vi "RT Status.vi"() -> ()   [LabVIEW 2019]
panel:
  out "rt queue":refnum<queue>
  out "status":string
  out "error out":errorcluster
  out "state":enum16{"connect", "run", "close"}(ring)
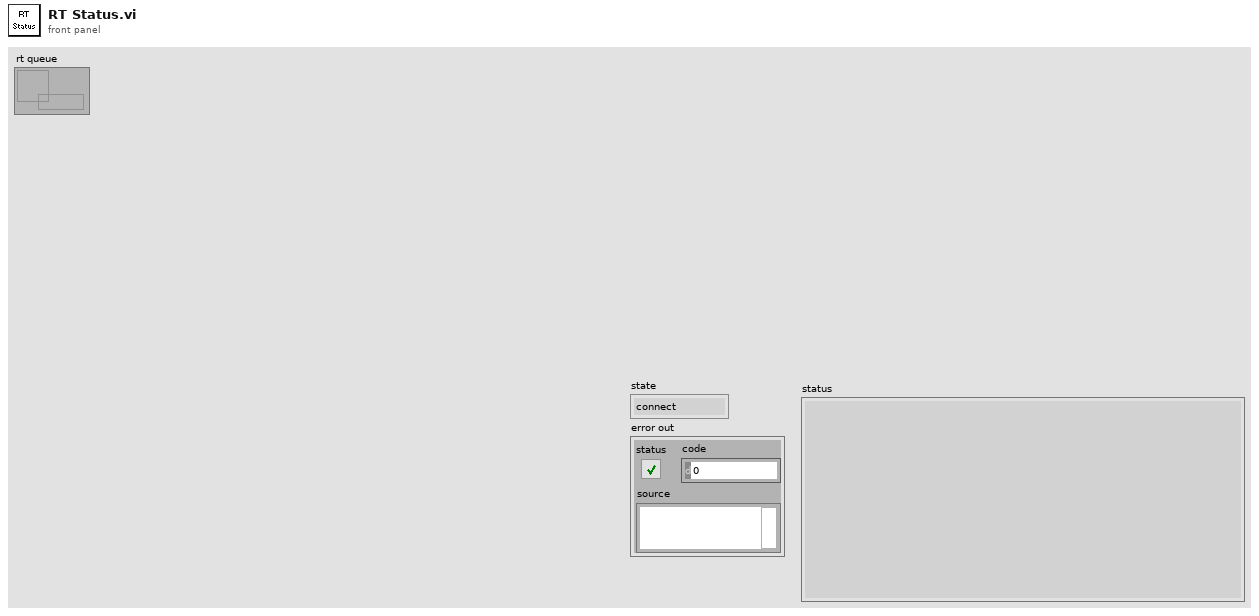
[diagram p1: front panel]
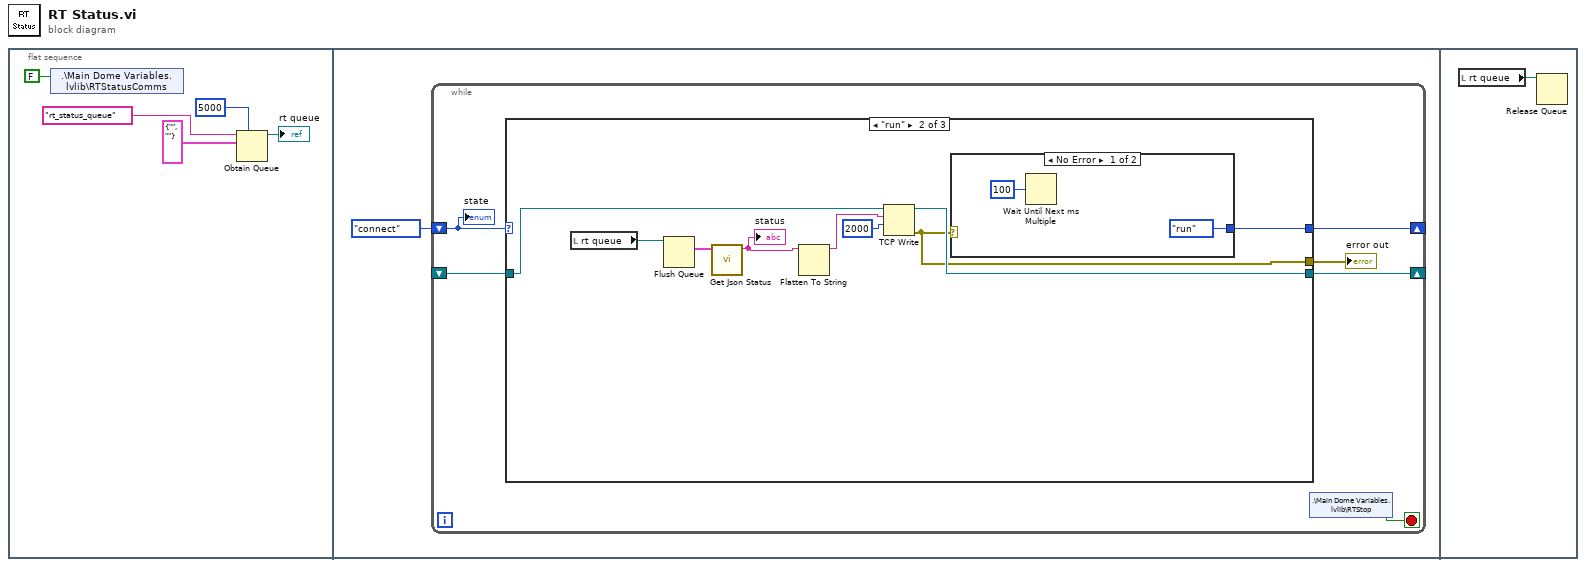
[diagram p0: block diagram]
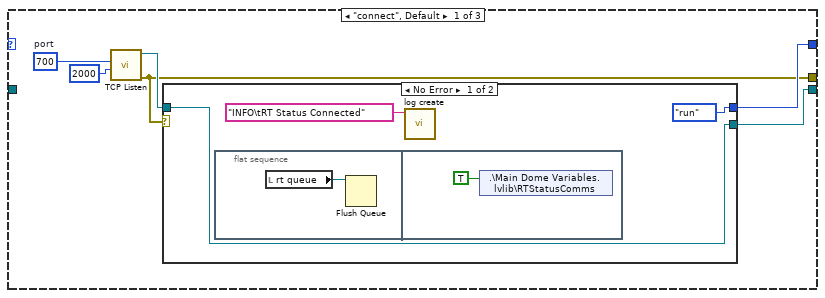
[diagram p2: hidden frame]
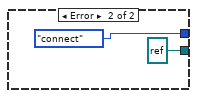
[diagram p3: hidden frame]
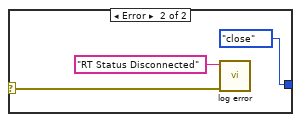
[diagram p4: hidden frame]
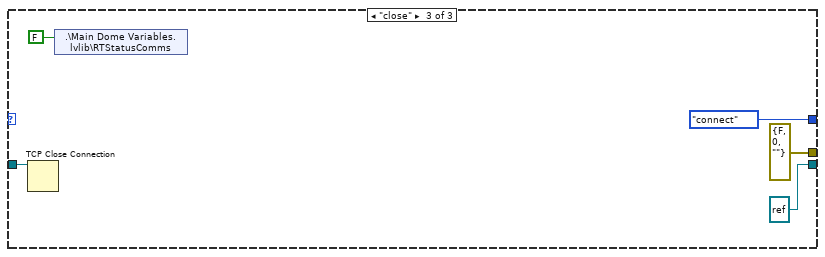
[diagram p5: hidden frame]
diagram:
  n1 = flat-sequence {
    frame #0 {
      n2 = shared-variable ".\\Main Dome Variables.lvlib\\RTStatusComms"(FALSE ("RTStatusComms")) -> ()  [unwired: 1 in, 1 out]
      n3 = Obtain Queue(max queue size (-1, unlimited)=5000, name (unnamed)="rt_status_queue", element data type=cluster{"time":string, "message":string} {"time"="", "message"=""}) -> (queue out=→"rt queue":refnum<queue>)  [unwired: 2 in, 2 out]
    }
    frame #1 {
      n4 = while {
        shift-right: [w10] -> _
        shift-left: enum16{"connect", "run", "close"}."connect" ("y") -> [w11]
        shift-right: [w9] -> _
        shift-left: _ -> [w8]
        stop <- w12 stop-if-true
        n5 = case shown="\"run\"" w11 {
          tunnel: [w16 w29 enum16{"connect", "run", "close"}."connect" ("y")] -> w10
          tunnel: [w15 w31 refnum<k5> refnum ("connection ID")] -> w9
          tunnel: w8 -> [_ w32 w42]
          tunnel: [w13 w28 errorcluster {"status"=FALSE, "code"=0, "source"=""} ("error out")] -> w7
          frame "connect", Default {
            w17 = u16 700  # port
            n6 = call <vilib>:"TCP Listen.vi"("timeout ms (wait forever: -1)"=2000, "port"=w17) -> ("error out"=w13:errorcluster, "connection ID"=w14:refnum<k5>)  [unwired: 2 in, 6 out]
            n7 = case shown="No Error" w13 {
              tunnel: [enum16{"connect", "run", "close"}."run" ("y") enum16{"connect", "run", "close"}."connect" ("y")] -> w16
              tunnel: [w20 refnum<k5> refnum ("connection ID")] -> w15
              tunnel: w14 -> [w20 _]
              frame No Error {
                n8 = flat-sequence {
                  frame #0 {
                    n9 = local read "rt queue"() -> (w22:refnum<queue>)
                    n10 = Flush Queue(queue=w22) -> ()  [unwired: 1 in, 3 out]
                  }
                  frame #1 {
                    n11 = shared-variable ".\\Main Dome Variables.lvlib\\RTStatusComms"(TRUE ("RTStatusComms")) -> ()  [unwired: 1 in, 1 out]
                  }
                }
                n12 = call "log create.vi"("message"="INFO\tRT Status Connected") -> ()  [unwired: 11 in]
              }
              frame Error {
              }
            }
          }
          frame "run" {
            n13 = local read "rt queue"() -> (w27:refnum<queue>)
            n14 = Flush Queue(queue=w27) -> (remaining elements=w26:cluster{"time":string, "message":string}[])  [unwired: 1 in, 2 out]
            n15 = call "Get Json Status.vi"("logger"=w26) -> ("out"=w34:string)  [unwired: 10 in]
            "status" <- w34
            n16 = Flatten To String(anything=w34) -> (data string=w33:string)  [unwired: 3 in, 2 out]
            n17 = TCP Write(connection ID=w32, data in=w33, 9:2000 ("timeout ms (25000)")) -> (connection ID out=w31:refnum<k5>, error out=w28:errorcluster)  [unwired: 1 in, 1 out]
            n18 = case shown="No Error" w28 {
              selector: w28 -> [_ w38]
              tunnel: [enum16{"connect", "run", "close"}."run" ("y") enum16{"connect", "run", "close"}."close" ("y")] -> w29
              frame No Error {
                n19 = Wait Until Next ms Multiple(millisecond multiple=u32 100) -> ()  [unwired: 1 out]
              }
              frame Error {
                n20 = call "log error.vi"("error in"=w38, "message"="RT Status Disconnected") -> ()  [unwired: 9 in, 1 out]
              }
            }
          }
          frame "close" {
            n21 = TCP Close Connection(connection ID=w42) -> ()  [unwired: 2 in, 2 out]
            n22 = shared-variable ".\\Main Dome Variables.lvlib\\RTStatusComms"(FALSE ("RTStatusComms")) -> ()  [unwired: 1 in, 1 out]
          }
        }
        "error out" <- w7
        n23 = shared-variable ".\\Main Dome Variables.lvlib\\RTStop"() -> (w12:bool)  [unwired: 1 in, 1 out]
        "state" <- w11
      }
    }
    frame #2 {
      n24 = local read "rt queue"() -> (w45:refnum<queue>)
      n25 = Release Queue(queue=w45) -> ()  [unwired: 2 in, 3 out]
    }
  }
